vi "CRYGet Tab in Table.vi"(9 "Legend":refnum<vi>, 10 "Mouse Point":T2, 11 "Table":refnum<vi>) -> (0 "bResult":bool, 1 "Cell Position":T1, 2 "Index":i32, 3 "Type":enum16{"Curves", "Values", "Results", "WFM"}(ring))   [LabVIEW 2013]
uses:
  <vilib>/Utility/miscctls.llb/LVPoint32TypeDef.ctl
  <vilib>/Utility/miscctls.llb/LVRowAndColumnTypeDef.ctl
  CRYCurveLibrary/Global/CRYCurve Library Global.vi
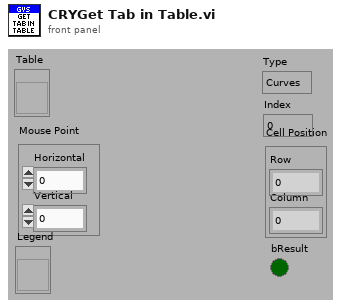
[diagram p1: front panel]
types:
  T1 = typedef "LVRowAndColumnTypeDef.ctl" = cluster{"Row":i32, "Column":i32}
  T2 = typedef "LVPoint32TypeDef.ctl" = cluster{"Horizontal":i32, "Vertical":i32}
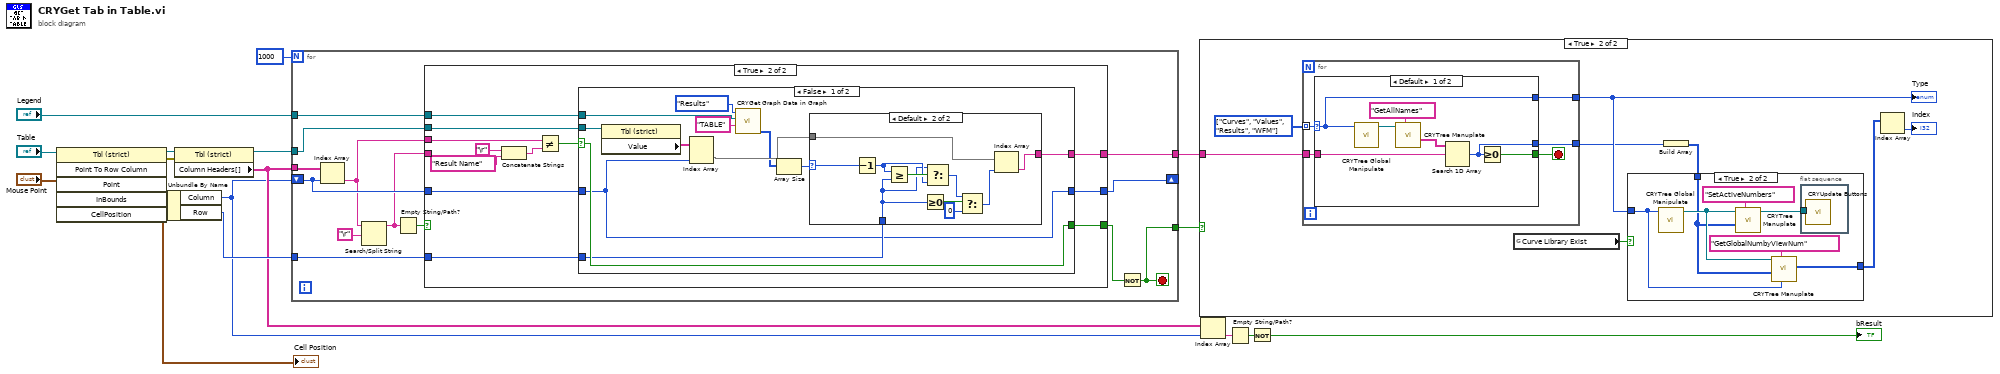
[diagram p0: block diagram]
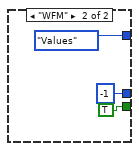
[diagram p4: hidden frame]
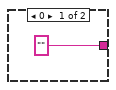
[diagram p6: hidden frame]
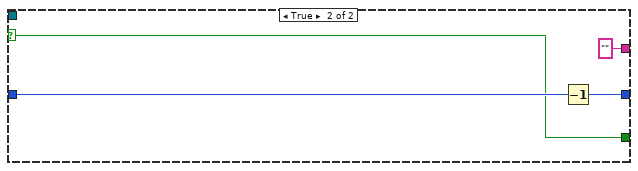
[diagram p7: hidden frame]
diagram:
  n1 = invoke class="Tbl (strict)" method="Point To Row Column"(reference="Table", "Point"="Mouse Point") -> (reference out=w14:refnum<vi>, error out=w13:errorcluster, "CellPosition"=w15:T1)  [unwired: 4 in, 3 out]
  "Cell Position" <- w15
  n2 = Unbundle By Name(w15) -> ("Column"=w1:i32, "Row"=w11:i32)
  n3 = property class="Tbl (strict)"(reference=w14, error in=w13) -> (reference out=w10:refnum<vi>, "Column Headers[]"=w5:string[])  [unwired: 1 out]
  n4 = for {
    N: 1000 -> [_]
    tunnel: w5 -> [w28]
    shift-right: [w25] -> _
    shift-left: w1 -> [w26]
    tunnel: [w21] -> w8
    tunnel: w11 -> [w20]
    tunnel: w10 -> [w19]
    tunnel: "Legend" -> [w18]
    tunnel: [w17] -> w6
    stop <- w17 stop-if-true
    n5 = Index Array(array=w28, index=w26) -> (element=w23:string)
    n6 = Search/Split String(string=w23, search string/char (-)="\r") -> (substring before match=w22:string)  [unwired: 3 out]
    n7 = Empty String/Path?(string/path=w22) -> (empty?=w27:bool)
    n8 = case shown="True" w27 {
      selector: w27 -> [w32 _]
      tunnel: [w32 w37] -> w24
      tunnel: w26 -> [w31 w44]
      tunnel: [w31 w43] -> w25
      tunnel: w23 -> [_ w42]
      tunnel: [w30 w34] -> w21
      tunnel: w22 -> [w30 _]
      tunnel: w20 -> [_ w36]
      tunnel: w19 -> [_ w35]
      tunnel: w18 -> [_ w33]
      frame False {
      }
      frame True {
        n9 = Concatenate Strings("\r", "Result Name" ("search string/char (-)")) -> (w39:string)
        n10 = Not Equal?(x=w42, y=w39) -> (x != y?=w38:bool)
        n11 = case shown="False" w38 {
          selector: w38 -> [w56 w69]
          tunnel: w44 -> [w51 w71]
          tunnel: [w51 w70] -> w43
          tunnel: [w56 w69] -> w37
          tunnel: w36 -> [w52 _]
          tunnel: w35 -> [w54 _]
          tunnel: [w55 ""] -> w34
          tunnel: w33 -> [w47 _]
          frame False {
            n12 = property class="Tbl (strict)"(reference=w54) -> ("Value"=w53:string[][])  [unwired: 1 in, 2 out]
            n13 = Index Array(array=w53, index (col)=w51) -> (element=w50:string[])  [unwired: 1 in]
            n14 = call "CRYGet Graph Data in Graph.vi"("Graph Type"="TABLE", "Legend Refnum"=w47, "Type In"=enum16{"Curves", "Values", "Results", "WFM"}."Results") -> ("Result Rows"=w46:i32[])  [unwired: 1 in, 7 out]
            n15 = Array Size(array=w46) -> (size(s)=w45:i32)
            n16 = case shown="Default" w45 {
              selector: w45 -> [_ w58]
              tunnel: ["" w67] -> w55
              tunnel: w52 -> [_ w63]
              tunnel: w50 -> [_ w66]
              frame 0 {
              }
              frame Default {
                n17 = Decrement(x=w58) -> (x-1=w64:i32)
                n18 = Greater Or Equal?(x=w64, y=w63) -> (x >= y?=w65:bool)
                n19 = Greater Or Equal To 0?(x=w63) -> (x >= 0?=w62:bool)
                n20 = Select(t=w63, s=w65, f=w64) -> (s? t:f=w61:i32)
                n21 = Select(t=w61, s=w62, f=0) -> (s? t:f=w59:i32)
                n22 = Index Array(array=w66, index=w59) -> (element=w67:string)
              }
            }
          }
          frame True {
            n23 = Decrement(x=w71) -> (x-1=w70:i32)
          }
        }
      }
    }
    n24 = Not(x=w24) -> (.not. x?=w17:bool)
  }
  n25 = case shown="True" w6 {
    tunnel: w8 -> [_ w75]
    frame False {
    }
    frame True {
      w78 = enum16{"Curves", "Values", "Results", "WFM"}[] [enum."Curves", enum."Values", enum."Results", enum."WFM"] items=["Curves", "Values", "Results", "WFM"]
      n26 = for {
        tunnel: w75 -> [w92]
        tunnel: w78 -> [w89] mode=indexing
        tunnel: [w88] -> w79
        tunnel: [w90] -> w77
        stop <- w91 stop-if-true
        n27 = case shown="Default" w89 {
          selector: w89 -> [w94 _]
          tunnel: w92 -> [w99 _]
          tunnel: [w98 TRUE] -> w91
          tunnel: [w97 -1 ("index of element")] -> w90
          tunnel: [w94 enum16{"Curves", "Values", "Results", "WFM"}."Values" ("Type")] -> w88
          frame Default {
            n28 = call "CRYTree Global Manipulate.vi"("Type In"=w94) -> ("Tree/Curve Tree"=w96:refnum<vi>)  [unwired: 7 in, 3 out]
            n29 = call "CRYTree Manuplate.vi"("sAction"="GetAllNames", "Tree in"=w96) -> ("sData Out"=w93:string[])  [unwired: 6 in, 3 out]
            n30 = Search 1D Array(1D array=w93, element=w99) -> (index of element=w97:i32)  [unwired: 1 out]
            n31 = Greater Or Equal To 0?(x=w97) -> (x >= 0?=w98:bool)
          }
          frame "WFM" {
          }
        }
      }
      "Type" <- w79
      n32 = global read "CRYCurve Library Global.vi" "Curve Library Exist"() -> (w74:bool)
      n33 = Build Array(w77) -> (w76:i32[])
      n34 = case shown="True" w74 {
        tunnel: w79 -> [_ w82]
        tunnel: w76 -> [w80 w84]
        tunnel: [w80 w83] -> w73
        frame False {
        }
        frame True {
          n35 = call "CRYTree Global Manipulate.vi"("Type In"=w82) -> ("Tree/Curve Tree"=w85:refnum<vi>)  [unwired: 7 in, 3 out]
          n36 = call "CRYTree Manuplate.vi"("sAction"="SetActiveNumbers", "nData"=w84, "Tree in"=w85) -> ("Tree Out"=w81:refnum<vi>)  [unwired: 5 in, 3 out]
          n37 = call "CRYTree Manuplate.vi"("Type"=w82, "sAction"="GetGlobalNumbyViewNum", "nData"=w84, "Tree in"=w85) -> ("nData Out"=w83:i32[])  [unwired: 4 in, 3 out]
          n38 = flat-sequence {
            tunnel: w81 -> [_]
            frame #0 {
              n39 = call "CRYUpdate Buttons.vi"() -> ()  [unwired: 12 in]
            }
          }
        }
      }
      n40 = Index Array(array=w73) -> (element=→"Index":i32)  [unwired: 1 in]
    }
  }
  n41 = Index Array(array=w5, index=w1) -> (element=w4:string)
  n42 = Empty String/Path?(string/path=w4) -> (empty?=w3:bool)
  n43 = Not(x=w3) -> (.not. x?=→"bResult":bool)
